vi "Messenger Initialize.vi"(7 "Elements Of Container":i32=-1, 8 "error in (no error)":errorcluster, 11 "Messenger Composite in":refnum<class "Tree-ArrayLocation Queue Messenger.lvclass">) -> (0 "error out":errorcluster, 3 "Messenger Composite out":refnum<class "Tree-ArrayLocation Queue Messenger.lvclass">)   [LabVIEW 2019, in "Tree-ArrayLocation Queue Messenger.lvclass"]
uses:
  Tree-ArrayLocation Queue Messenger.lvclass
  Ancestor Class/Message/Message.lvclass
  Tree-ArrayLocation Queue Messenger.lvclass/Tree-ArrayLocation Queue Messenger.ctl
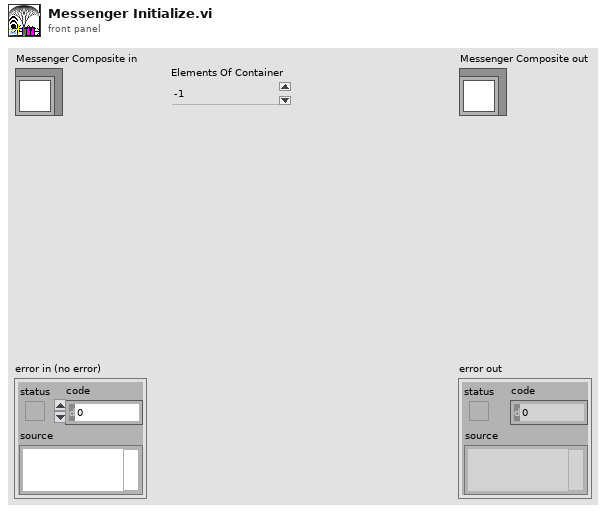
[diagram p1: front panel]
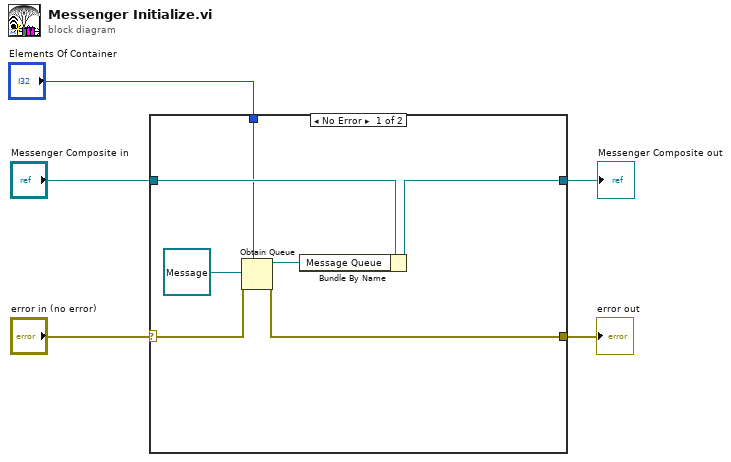
[diagram p0: block diagram]
diagram:
  n1 = case shown="No Error" "error in (no error)" {
    selector: "error in (no error)" -> [w8 w14]
    tunnel: [w7 w14] -> w4
    tunnel: [w9 w13] -> w3
    tunnel: "Messenger Composite in" -> [w11 w13]
    tunnel: "Elements Of Container" -> [w6 _]
    frame No Error {
      n2 = Obtain Queue(max queue size (-1, unlimited)=w6, element data type=refnum<class "Message.lvclass"> refnum ("Message.lvclass"), error in (no error)=w8) -> (queue out=w10:refnum<queue>, error out=w7:errorcluster)  [unwired: 2 in, 1 out]
      n3 = Bundle By Name(cluster=w11, "Message Queue"=w10) -> (w9:refnum<class "Tree-ArrayLocation Queue Messenger.lvclass">)
    }
    frame Error {
    }
  }
  "error out" <- w4
  "Messenger Composite out" <- w3
